vi "VI 1.vi"() -> ()   [LabVIEW 2017]
panel:
  out "String":string="Try GitHub"
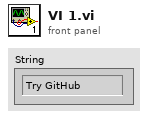
[diagram p1: front panel]
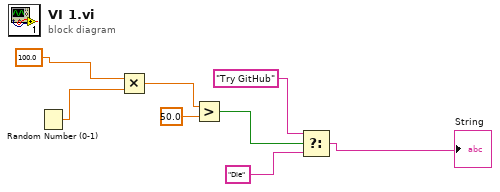
[diagram p0: block diagram]
diagram:
  n1 = Random Number (0-1)() -> (number: 0 to 1=w8:dbl)
  n2 = Multiply(x=100.0, y=w8) -> (x*y=w5:dbl)
  n3 = Greater?(x=w5, y=50.0) -> (0:w4:bool)
  n4 = Select(t="Try GitHub", s=w4, f="Die") -> (s? t:f=→"String":string)
